vi "Get Fail Code.vi"(8 "error in (no error)":errorcluster, 11 "Test Class in":refnum<class "Test Class.lvclass">) -> (0 "error out":errorcluster, 2 "Fail Code":string)   [LabVIEW 2015, in "Test Class.lvclass"]
uses:
  Test Class.lvclass
  Test Class.lvclass/Test Class.ctl
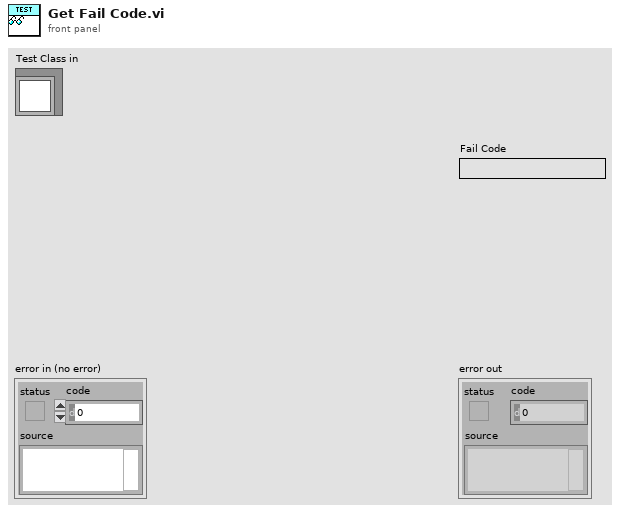
[diagram p1: front panel]
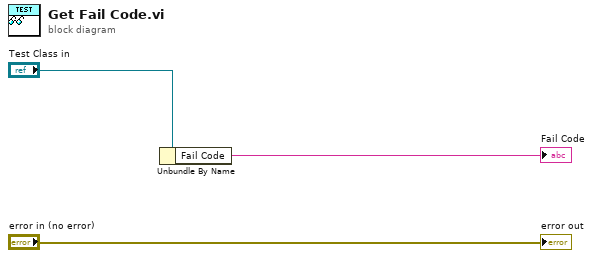
[diagram p0: block diagram]
diagram:
  n1 = Unbundle By Name("Test Class in") -> ("Fail Code"=→"Fail Code":string)
  "error out" <- "error in (no error)"
